vi "data change.vi"(6 "Module ID":i32=-1, 8 "error in":errorcluster, 9 "changed data":string, 10 "view number":i32, 11 "view name":string) -> (0 "error out":errorcluster)   [LabVIEW 2022 SP3, in "Model Thread.lvlib"]
doc: "_____\nCreated using DQMH Event Scripter 6.1.0.128."
uses:
  Model Thread.lvlib
  data change Argument--cluster.ctl
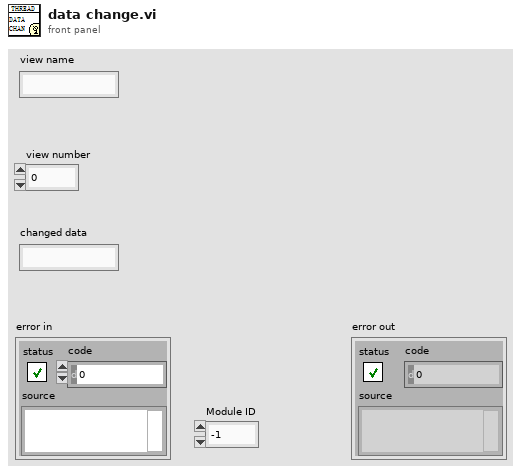
[diagram p1: front panel]
types:
  T1 = typedef "Model Thread.lvlib/data change Argument--cluster.ctl" = cluster{"Module ID":i32, "view number":i32, "view name":string, "changed data":string}
  T2 = typedef "Model Thread.lvlib/Broadcast Events--cluster.ctl" = cluster{"Module Did Init":refnum<user-event>, "Status Updated":refnum<user-event>, "Error Reported":refnum<user-event>, "Module Did Stop":refnum<user-event>, "Update Module Execution Status":refnum<user-event>, "data change":refnum<user-event>}
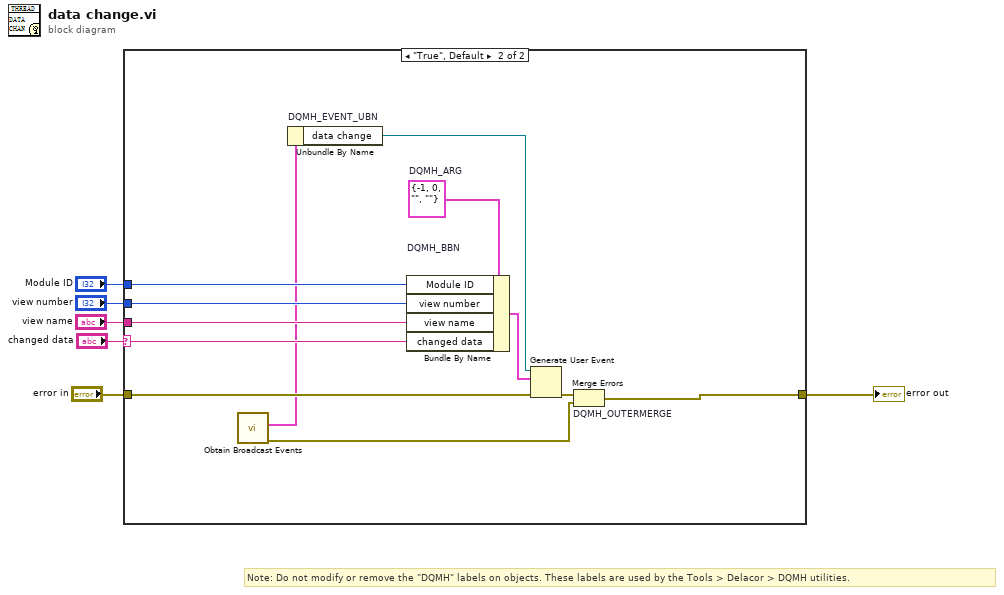
[diagram p0: block diagram]
diagram:
  # "Note: Do not modify or remove the \"DQMH\" labels on objects. These labels are used by the Tools > Delacor > DQMH utilities."
  n1 = case shown="\"True\", Default" "changed data" {
    selector: "changed data" -> [_ w9]
    tunnel: [w7 w19] -> w6
    tunnel: "error in" -> [w7 w18]
    tunnel: "Module ID" -> [_ w13]
    tunnel: "view number" -> [_ w12]
    tunnel: "view name" -> [_ w11]
    frame "" {
    }
    frame "True", Default {
      w14 = T1 {"Module ID"=-1, "view number"=0, "view name"="", "changed data"=""}  # DQMH_ARG
      n2 = call "Obtain Broadcast Events.vi"() -> ("error out"=w10:errorcluster, "Model Thread Broadcast Events"=w8:T2)  [unwired: 10 in]
      n3 = Unbundle By Name "DQMH_EVENT_UBN"(w8) -> ("data change"=w16:refnum<user-event>)
      n4 = Bundle By Name "DQMH_BBN"(cluster=w14, "Module ID"=w13, "view number"=w12, "view name"=w11, "changed data"=w9) -> (w17:T1)
      n5 = Generate User Event(user event=w16, event data cluster=w17, error in=w18) -> (error out=w15:errorcluster)  [unwired: 1 in, 1 out]
      n6 = Merge Errors "DQMH_OUTERMERGE"(w15, w10) -> (w19:errorcluster)
    }
  }
  "error out" <- w6
